vi "sccx.vi"(6 "DLLPath":path, 8 "error in (no error)":errorcluster, 9 "SCCX Parameters":T2={"I_Range"=11, "E_Range"=0, "Bandwidth"=3, "par_E0"=1.0, "par_A"=0.0, "par_B"=0.1, "par_QRP_select"=1, "par_E_duration"=0.01, "par_E_dt_rec"=0.0001, "par_I0_duration"=0.01, "par_I0_dt_rec"=0.0001, "par_NC"=9, "par_RC"=1, "par_Q_limit_val"=5e-05, "par_Q_limit_cfg"=0, "par_QRP_time"=0.005, "ce"=0, "em"=0} {"par_Q_limit_cfg" items=["Disable"=0, "Enable if <"=129, "Enable if >"=133]; "par_QRP_select" items=["Ewe", "Ece"]; "E_Range" items=["±2.5V", "±5V", "±10V", "Auto"]; "Bandwidth" items=["1"=1, "2"=2, "3"=3, "4"=4, "5"=5, "6"=6, "7"=7, "8"=8, "9"=9]; "I_Range" items=["1pA", "1nA", "10nA", "100nA", "1µA", "10µA", "100µA", "1mA", "10mA", "100mA", "1A", "Booster", "Auto"]}, 10 "Channel":u8(ring) items=["1", "2", "3", "4", "5", "6", "7", "8", "9", "10", "11", "12", "13", "14", "15", "16"], 11 "IP adress":string="192.109.209.229") -> (0 "error out":errorcluster, 1 "XY Graph":cluster{"Data 101":sgl[], "Data 101":sgl[]}(graph), 2 "Output Data":T1, 3 "Exit 2":bool=TRUE)   [LabVIEW 2022 SP3]
doc: "Chrono-Amperometry (CA) is a controlled-potential technique. The current response is measured to an applied potential step.\nIn general, in this VI, the first thing to do is to start by establishing the connection with the instrument defined by its IP adress, then load the firmware in the channel selected, get the information on the plugged channels, load protocol on a channel, start/stop the protocol, retreive data and draw the graph."
uses:
  Library/EClib Functions/SCCXParameters.ctl
  Library/EClib Functions/Parameters.ctl
  Library/EClib Functions/EClib functions.lvlib
panel:
  in  "Display Parameters?":bool caption="Display Parameters"
  out "DllPath":path caption="DLL Path"
  out "LibVersion":string caption="DLL Version"
  in  "Draw":enum16{"Ewe(t)", "Ece(t)", "I(t)", "Q(t)"}(ring)
  out "Number of points":i32=1992
  out "Data 174":sgl[][](array[numeric]) format="%.2f"
  in  "stop":bool
  in  "Exit":bool
  in  "Start":bool
  # "Instructions:\nBefore running the VI you must type a valid IP adress that corresponds to the instrument.Then press the Run button to execute this VI.\nWhile this VI is running, choose the available channel, enter the CA parameters or keep the default values, then press the start button to begin the experience.\nChoose the waveform to draw (Ewe(t) or I(t)). You can stop the measure if you press the stop button and exit the execution if you press the exit button."
  # "V"
  # "Next En+1 = En - B * (A - QRP)"
  # "s"
  # "s"
  # "Switch to  I = 0"
  # "s"
  # "s"
  # "s"
  # "C"
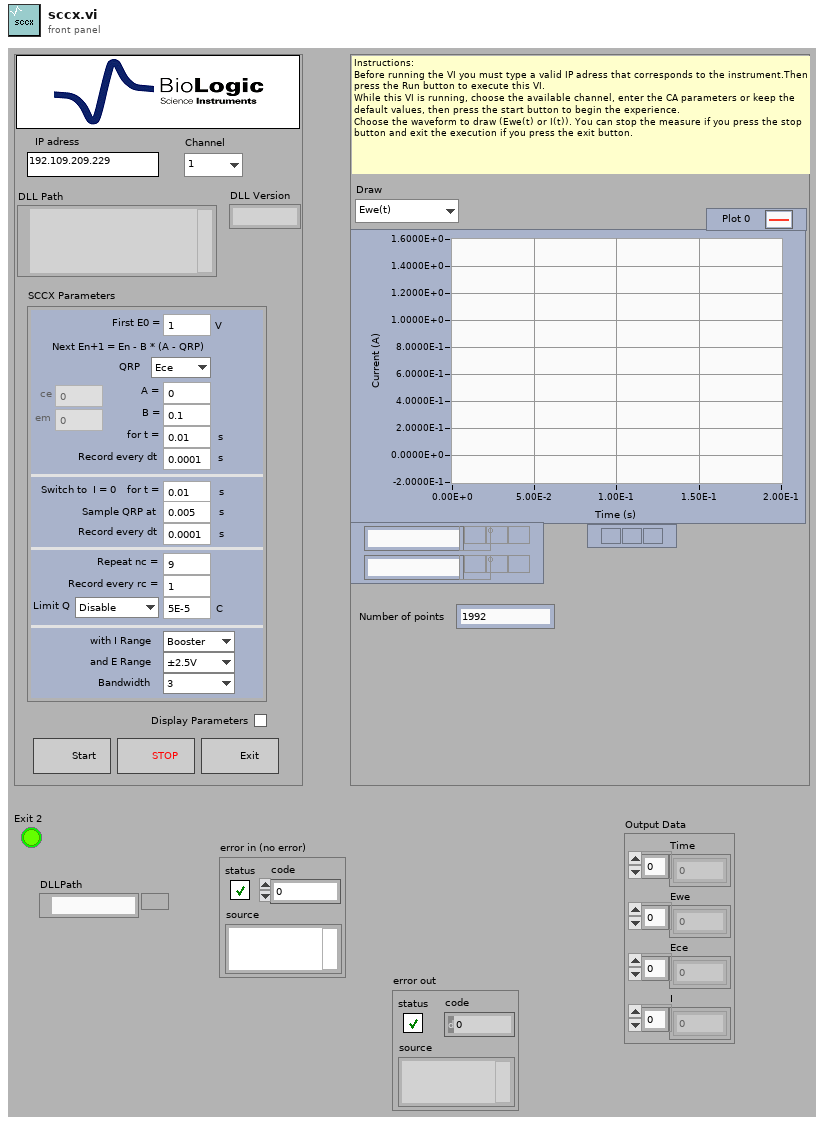
[diagram p1: front panel]
types:
  T1 = cluster{"Time":sgl[], "Ewe":sgl[], "Ece":sgl[], "I":sgl[]}
  T2 = typedef "EClib functions.lvlib/SCCXParameters.ctl" = cluster{"I_Range":u16, "E_Range":u16, "Bandwidth":u16, "par_E0":sgl, "par_A":sgl, "par_B":sgl, "par_QRP_select":u16, "par_E_duration":sgl, "par_E_dt_rec":sgl, "par_I0_duration":sgl, "par_I0_dt_rec":sgl, "par_NC":i32, "par_RC":i32, "par_Q_limit_val":sgl, "par_Q_limit_cfg":u16, "par_QRP_time":sgl, "ce":i32, "em":i32}
  T3 = cluster{"LibVersion":string, "StringLength":u32, "DllPath":path}
  T4 = cluster{"Channel":i32, "BoardVersion":i32, "BoardSerialCode":i32, "FirmwareCode":i32, "FirmwareVersion":i32, "XilinxVersion":i32, "AmpCode":i32, "NbAmp":i32, "LcBoard":i32, "Zboard":i32, "MuxBoard":i32, "GPRAboard":i32, "MemSize":i32, "MemFilled":i32, "state":i32, "MaxIRange":i32, "MinIRange":i32, "MaxBandwidth":i32, "NbOfTechniques":i32}
  T5 = typedef "EClib functions.lvlib/Parameters.ctl" = enum16{"CA", "CASG", "CP", "GEIS", "ISCAN", "OCV", "PEIS", "SCCX", "SGEIS", "SPEIS", "VSCAN", "MP"}
  T6 = cluster{"SCCX Parameters":T2, "Channel information":cluster{"Channel":i32, "BoardVersion":i32, "BoardSerialCode":i32, "FirmwareCode":i32, "FirmwareVersion":i32, "XilinxVersion":i32, "AmpCode":i32, "NbAmp":i32, "LcBoard":i32, "Zboard":i32, "MuxBoard":i32, "GPRAboard":i32, "MemSize":i32, "MemFilled":i32, "state":i32, "MaxIRange":i32, "MinIRange":i32, "MaxBandwidth":i32, "NbOfTechniques":i32}}
  T7 = typedef "EClib functions.lvlib/TechniqueParameters.ctl" = cluster{"String Label":string, "Type":i32, "Valeur":i32, "Index":i32}
  T8 = cluster{"string before end tag":string, i32, i32, i32}[]
  T9 = cluster{"IRQskipped":i32, "NbRaws":i32, "NbCols":i32, "Technique Index":i32, "TechniqueID":i32, "PrcessIndex":i32, "loop":i32, "StartTime":dbl, "MuxPad":i32}
  T10 = cluster{"State":i32, "MemFilled":i32, "TimeBase":sgl, " Ewe":sgl, " EweRangeMin":sgl, " EweRangeMax":sgl, "Ece":sgl, "EceRangeMin":sgl, "EceRangeMax":sgl, "Eoverflow":i32, "I":sgl, "IRange":i32, "Ioverflow":i32, "ElapsedTime":sgl, "Freq":sgl, "Rcomp":sgl, "Saturation":sgl, "OptErr":i32, "OptPos":i32}
  T11 = cluster{"Data 174":sgl[], "Data 174":sgl[], "Data 174":sgl[], "Data 174":sgl[]}
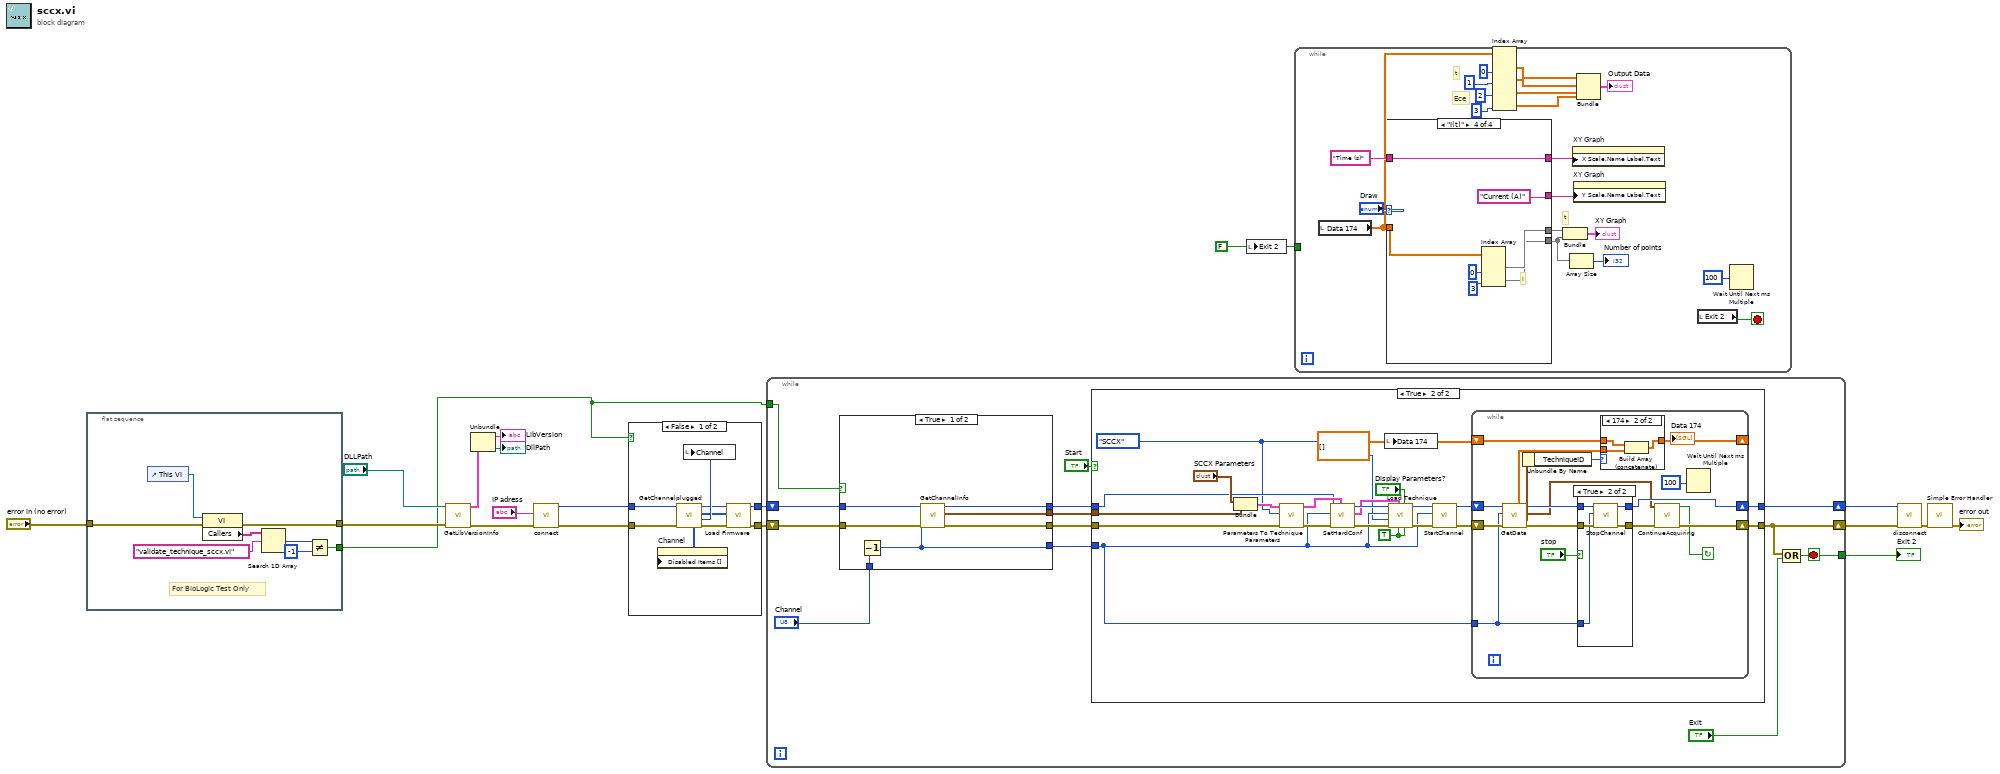
[diagram p0: block diagram]
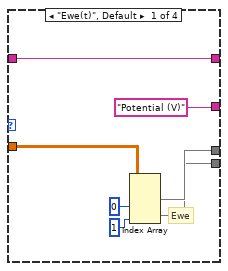
[diagram p3: hidden frame]
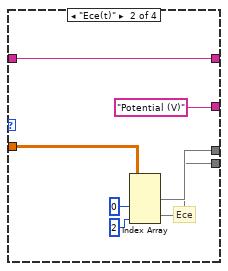
[diagram p4: hidden frame]
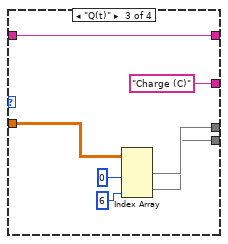
[diagram p5: hidden frame]
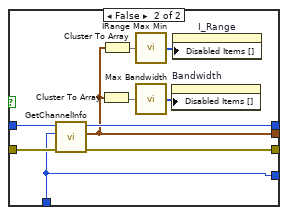
[diagram p6: hidden frame]
diagram:
  w18 = FALSE ("Exit 2")
  n1 = flat-sequence {
    tunnel: "error in (no error)" -> [w26]
    tunnel: [w25] -> w2
    tunnel: [w20] -> w1
    frame #0 {
      # "For BioLogic Test Only"
      n2 = control-ref of="This VI"() -> (w27:refnum<vi>)
      n3 = property class="VI"(reference=w27, error in=w26) -> (error out=w25:errorcluster, "Callers"=w24:string[])  [unwired: 1 out]
      n4 = Search 1D Array(1D array=w24, element="validate_technique_sccx.vi") -> (index of element=w22:i32)  [unwired: 1 in]
      n5 = Not Equal?(x=w22, y=-1) -> (x != y?=w20:bool)
    }
  }
  n6 = call "GetLibVersionInfo.vi"("error in (no error)"=w2, "DLLPath"="DLLPath") -> ("error out"=w6:errorcluster, "LibInfo"=w9:T3)  [unwired: 8 in]
  n7 = Unbundle(w9) -> ("LibVersion"=→"LibVersion":string, "DllPath"=→"DllPath":path)  [unwired: 1 out]
  n8 = call "connect.vi"("error in (no error)"=w6, "IP"="IP adress") -> ("error out"=w16:errorcluster, "ID Out"=w14:i32)  [unwired: 5 in, 3 out]
  n9 = case shown="False" w1 {
    tunnel: w16 -> [w35 w37]
    tunnel: [w33 w37] -> w15
    tunnel: w14 -> [w30 w38]
    tunnel: [w29 w38] -> w13
    frame False {
      n10 = call "GetChannelplugged.vi"("error in (no error)"=w35, "ID In"=w30) -> ("error out"=w32:errorcluster, "FirstPluggedChannel"=w36:u8, "PluggedChannels"=w28:u8[], "ID Out"=w31:i32, "DisabledChannels"=w34:i32[])  [unwired: 5 in]
      n11 = property on="Channel" class="Ring (strict)"("Disabled Items []"=w34) -> ()  [unwired: 2 in, 2 out]
      n12 = local write "Channel"(w36) -> ()
      n13 = call "Load Firmware.vi"("error in (no error)"=w32, "Channels"=w28, "ID In"=w31) -> ("error out"=w33:errorcluster, "ID Out"=w29:i32)  [unwired: 6 in, 1 out]
    }
    frame True {
    }
  }
  n14 = while {
    shift-right: [w43] -> w12
    shift-left: w15 -> [w50]
    tunnel: [w41] -> w19
    shift-right: [w45] -> w11
    shift-left: w13 -> [w47]
    tunnel: w1 -> [w40]
    stop <- w41 stop-if-true
    n15 = case shown="True" w40 {
      tunnel: w50 -> [w58 w64]
      tunnel: [w57 w63] -> w49
      tunnel: "Channel" -> [w53 w59]
      tunnel: w47 -> [w56 w62]
      tunnel: [w55 w61] -> w46
      tunnel: [w54 w60] -> w44
      tunnel: [w52 w59] -> w39
      frame True {
        n16 = Decrement(x=w53) -> (x-1=w52:u8)
        n17 = call "GetChannelInfo.vi"("error in (no error)"=w58, "Channel"=w52, "ID"=w56) -> ("error out"=w57:errorcluster, "Channel information"=w54:T4, "ID Out"=w55:i32)  [unwired: 6 in]
      }
      frame False {
        n18 = call "GetChannelInfo.vi"("error in (no error)"=w64, "Channel"=w59, "ID"=w62) -> ("error out"=w63:errorcluster, "Channel information"=w60:T4, "ID Out"=w61:i32)  [unwired: 6 in]
        n19 = Cluster To Array(cluster=w60) -> (array=w67:i32[])
        n20 = Cluster To Array(cluster=w60) -> (array=w68:i32[])
        n21 = call "IRange Max Min.vi"("resources"=w68) -> ("disabled ranges"=w65:i32[])
        n22 = call "Max Bandwidth.vi"("resources"=w67) -> ("disabled ranges"=w66:i32[])
        n23 = property on="Bandwidth" class="Ring (strict)"("Disabled Items []"=w66) -> ()  [unwired: 2 in, 2 out]
        n24 = property on="I_Range" class="Ring (strict)"("Disabled Items []"=w65) -> ()  [unwired: 2 in, 2 out]
      }
    }
    n25 = case shown="True" "Start" {
      tunnel: [w70 w91] -> w43
      tunnel: w49 -> [w70 w73]
      tunnel: w46 -> [w69 w72]
      tunnel: [w69 w84] -> w45
      tunnel: w44 -> [_ w77]
      tunnel: w39 -> [_ w74]
      frame False {
      }
      frame True {
        w71 = Parameters."SCCX" ("Parameters")
        w88 = TRUE ("First Protocol")
        w90 = sgl[][] []
        n26 = Bundle("SCCX Parameters"="SCCX Parameters", "Channel information"=w77) -> (w75:T6)  [unwired: 1 in]
        n27 = call "Parameters To Technique Parameters.vi"("error in (no error)"=w73, "Parameters"=w71, "ParameterIN"=w75) -> ("error out"=w83:errorcluster, "Params Values"=w79:T7[])  [unwired: 7 in]
        n28 = call "SetHardConf.vi"("Params Values"=w79, "error in (no error)"=w83, "Channel"=w74, "ID In"=w72) -> ("error out"=w82:errorcluster, "Params Values Trimed"=w80:T8, "ID Out"=w81:i32)  [unwired: 5 in]
        n29 = local write "Data 174"(w90) -> ()
        n30 = call "Load Technique.vi"("Last Protocol"=w88, "Display Parameters?"="Display Parameters?", "First Protocol"=w88, "TechniqueParameters"=w80, "error in (no error)"=w82, "Parameters"=w71, "Selected Channel"=w74, "ID In"=w81) -> ("error out"=w87:errorcluster, "ID  Out"=w86:i32)  [unwired: 1 in, 1 out]
        n31 = call "StartChannel.vi"("error in (no error)"=w87, "Channel"=w74, "ID In"=w86) -> ("error out"=w89:errorcluster, "ID Out"=w85:i32)  [unwired: 7 in]
        n32 = while {
          shift-right: [w96] -> w91
          shift-left: w89 -> [w108]
          shift-right: [w105] -> _
          shift-left: w90 -> [w106]
          shift-right: [w97] -> w84
          shift-left: w85 -> [w99]
          tunnel: w74 -> [w92]
          stop <- w93 continue-if-true
          n33 = call "GetData.vi"("error in (no error)"=w108, "Channel"=w92, "ID In"=w99) -> ("error out"=w104:errorcluster, "Data information"=w102:T9, "Current values"=w94:T10, "ID Out"=w98:i32, "Data"=w100:dbl[][])  [unwired: 1 in, 3 out]
          n34 = Unbundle By Name(w102) -> ("TechniqueID"=w101:i32)
          n35 = case shown="True" "stop" {
            tunnel: [w110 w115] -> w95
            tunnel: w104 -> [w110 w114]
            tunnel: w98 -> [w109 w113]
            tunnel: [w109 w112] -> w97
            tunnel: w92 -> [_ w111]
            frame False {
            }
            frame True {
              n36 = call "StopChannel.vi"("error in (no error)"=w114, "Channel"=w111, "ID In"=w113) -> ("error out"=w115:errorcluster, "ID Out"=w112:i32)  [unwired: 7 in]
            }
          }
          n37 = case shown="174" w101 {
            tunnel: w100 -> [_ w119]
            tunnel: w106 -> [w116 w118]
            tunnel: [w116 w117] -> w105
            frame 0, Default {
            }
            frame 174 {
              n38 = Build Array (concatenate)(w118, w119) -> (w117:dbl[][])
            }
          }
          "Data 174" <- w105
          n39 = call "ContinueAcquiring.vi"("error in"=w95, "Current values"=w94) -> ("error out"=w96:errorcluster, "ContinueAcquiring?"=w93:bool)  [unwired: 8 in]
          n40 = Wait Until Next ms Multiple(millisecond multiple=u32 100) -> ()  [unwired: 1 out]
        }
      }
    }
    n41 = Compound Arithmetic op=OR(w43, "Exit") -> (w41:bool)
  }
  "Exit 2" <- w19
  n42 = local write "Exit 2"(w18) -> ()
  n43 = while {
    tunnel: w18 -> [_]
    stop <- w138 stop-if-true
    # "Ece"
    # "t"
    # "t"
    n44 = local read "Data 174"() -> (w124:sgl[][])
    n45 = case shown="\"I(t)\"" "Draw" {
      tunnel: ["Potential (V)" ("Y Scale.Name Label.Text") "Potential (V)" ("Y Scale.Name Label.Text") "Charge (C)" ("Y Scale.Name Label.Text") "Current (A)" ("Y Scale.Name Label.Text")] -> w136
      tunnel: [w146 w153 w160 w167] -> w135
      tunnel: "Time (s)" ("Y Scale.Name Label.Text") -> [w146 w153 w160 w167]
      tunnel: w124 -> [w143 w150 w158 w164]
      tunnel: [w141 w148 w155 w162] -> w132
      tunnel: [w140 w147 w154 w161] -> w131
      frame "Ewe(t)", Default {
        # "Ewe"
        n46 = Index Array(array=w143, index (col) #1=0 ("Index"), index (col) #2=1 ("Index")) -> (element #1=w141:sgl[], element #2=w140:sgl[])  [unwired: 2 in]
      }
      frame "Ece(t)" {
        # "Ece"
        n47 = Index Array(array=w150, index (col) #1=0 ("Index"), index (col) #2=2 ("Index")) -> (element #1=w148:sgl[], element #2=w147:sgl[])  [unwired: 2 in]
      }
      frame "Q(t)" {
        n48 = Index Array(array=w158, index (col) #1=0 ("Index"), index (col) #2=6 ("indice désactivé (col)")) -> (element #1=w155:sgl[], element #2=w154:sgl[])  [unwired: 2 in]
      }
      frame "I(t)" {
        # "I"
        n49 = Index Array(array=w164, index (col) #1=0 ("Index"), index (col) #2=3 ("indice désactivé (col)")) -> (element #1=w162:sgl[], element #2=w161:sgl[])  [unwired: 2 in]
      }
    }
    n50 = Index Array(array=w124, index (col) #1=0 ("Index"), index (col) #2=1 ("indice désactivé (col)"), index (col) #3=2 ("index (col)"), index (col) #4=3 ("index (col)")) -> (element #1=w123:sgl[], element #2=w122:sgl[], element #3=w121:sgl[], element #4=w120:sgl[])  [unwired: 4 in]
    n51 = Bundle("Data 174"=w132, "Data 174"=w131) -> (→"XY Graph":cluster{"Data 174":sgl[], "Data 174":sgl[]})  [unwired: 1 in]
    n52 = Array Size(array=w131) -> (size(s)=→"Number of points":i32)
    n53 = property on="XY Graph" class="XYGraph (strict)"("X Scale.Name Label.Text"=w135) -> ()  [unwired: 2 in, 2 out]
    n54 = property on="XY Graph" class="XYGraph (strict)"("Y Scale.Name Label.Text"=w136) -> ()  [unwired: 2 in, 2 out]
    n55 = Bundle("Data 174"=w123, "Data 174"=w122, "Data 174"=w121, "Data 174"=w120) -> (→"Output Data":T11)  [unwired: 1 in]
    n56 = local read "Exit 2"() -> (w138:bool)
    n57 = Wait Until Next ms Multiple(millisecond multiple=u32 100) -> ()  [unwired: 1 out]
  }
  n58 = call "disconnect.vi"("error in (no error)"=w12, "ID In"=w11) -> ("error out"=w10:errorcluster)  [unwired: 9 in]
  n59 = call <vilib>:"Simple Error Handler.vi"("error in (no error)"=w10) -> ("error out"=→"error out":errorcluster)  [unwired: 4 in, 4 out]
